vi "Encrypt.vi"(8 "error in (no error)":errorcluster, 10 "Plaintext":string, 11 "AES in":refnum<class "AES.lvclass">) -> (0 "error out":errorcluster, 2 "Cyphertext":string, 3 "AES out":refnum<class "AES.lvclass">)   [LabVIEW 2020, in "AES.lvclass"]
uses:
  AES.lvclass
  AES.lvclass/AES.ctl
  Ton Plomp Encryption/Encryption.lvlib
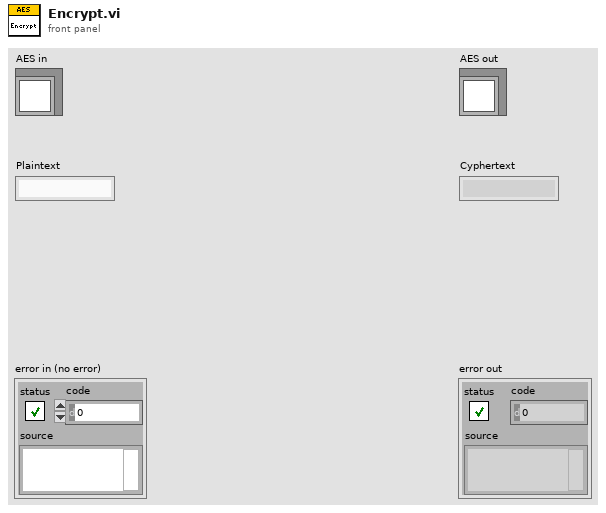
[diagram p1: front panel]
types:
  T1 = typedef "Encryption.lvlib/AES-Modes.ctl" = enum16{"ECB", "CBC", "CFB128", "OFB"}
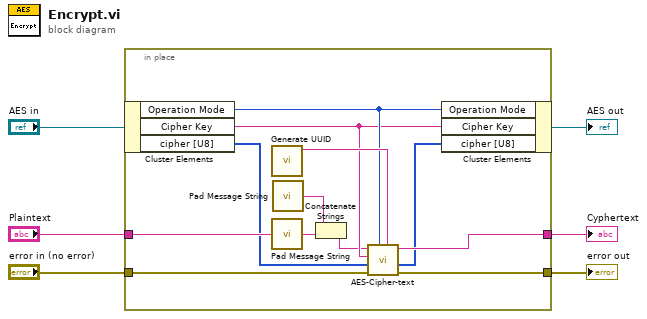
[diagram p0: block diagram]
diagram:
  n1 = in-place {
    in-place-border: "error in (no error)" -> [w15]
    in-place-border: [w14] -> w3
    in-place-border: [w12] -> w2
    in-place-border: "Plaintext" -> [w13]
    n2 = in-place-cluster #1("AES in") -> ("Operation Mode"=w17:T1, "Cipher Key"=w16:string, "cipher [U8]"=w9:u8[])
    n3 = call "Generate UUID.vi"() -> ("String UUID"=w18:string)  [unwired: 9 in, 2 out]
    n4 = call "Pad Message String.vi"("Message In"=w13) -> ("Padded Message Out"=w10:string)
    n5 = call "Pad Message String.vi"() -> ("Padded Message Out"=w7:string)  [unwired: 1 in]
    n6 = Concatenate Strings(w7, w10) -> (w11:string)
    n7 = call "AES-Cipher-text.vi"("Initializer Vector"=w18, "Operation Mode"=w17, "error in (no error)"=w15, "cipher [U8]"=w9, "Cipher Key"=w16, "Message in"=w11) -> ("error out"=w14:errorcluster, "cipher out"=w8:u8[], "Ciphered message"=w12:string)  [unwired: 3 in]
    n8 = in-place-cluster #1("Operation Mode"=w17, "Cipher Key"=w16, "cipher [U8]"=w8) -> (→"AES out":refnum<class "AES.lvclass">)
  }
  "error out" <- w3
  "Cyphertext" <- w2
